vi "Read TDMS.vi"(6 "Append Index":i32, 8 "error in (no error)":errorcluster, 11 "path":path) -> (0 "error out":errorcluster, 1 "Commands":string, 2 "Notes":string, 3 "Data (Dictionary)":T1[](array[typedef]))   [LabVIEW 2016, in "LV-Data.TDMS.lvclass"]
uses:
  LV-Data.TDMS.lvclass
  LV-Data/Typedefs/Dictionary--cluster.ctl
  LV-Data/LV-Data.lvclass
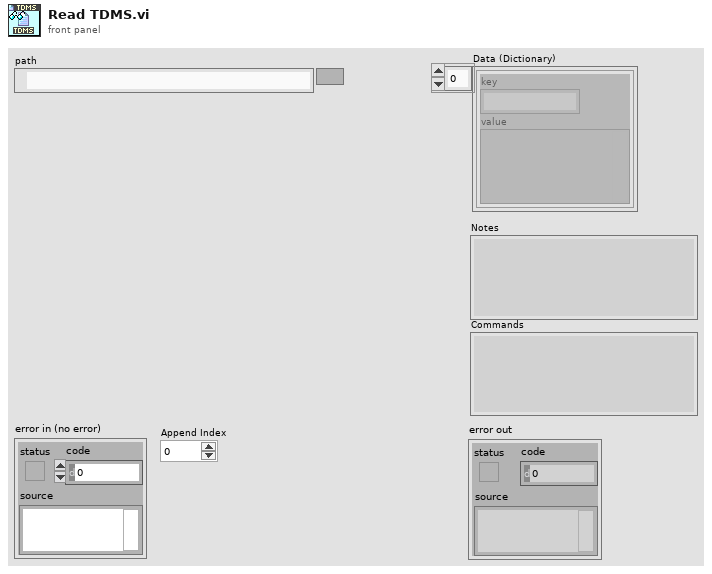
[diagram p1: front panel]
types:
  T1 = typedef "LV-Data.lvclass/Dictionary--cluster.ctl" = cluster{"key":string, "value":variant}
  T2 = enum16{"open", "open or create", "create or replace", "create", "open (read-only)"}
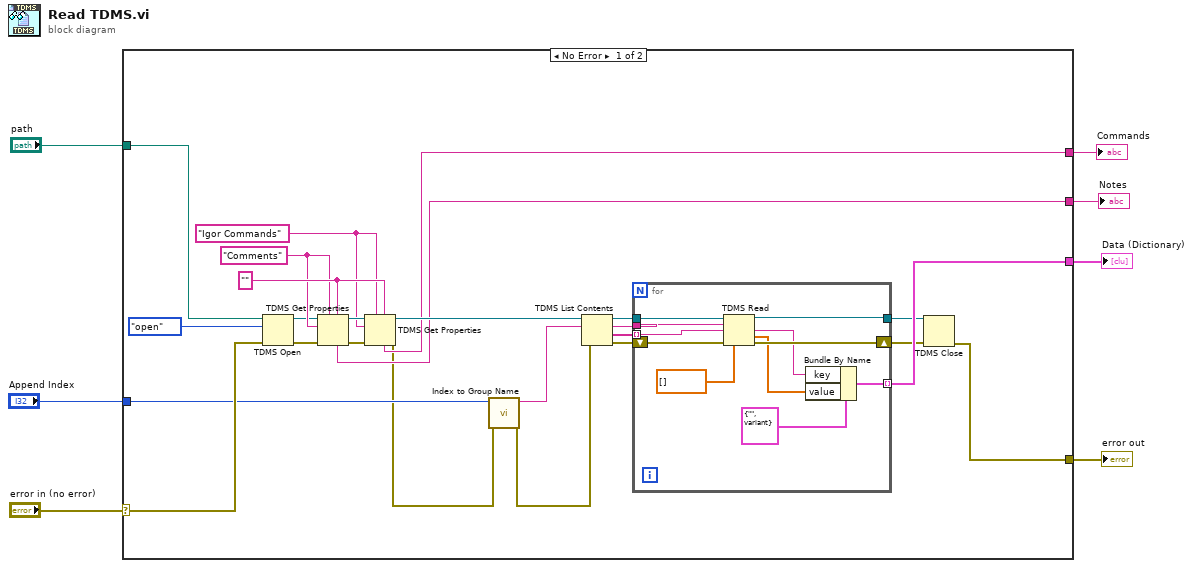
[diagram p0: block diagram]
diagram:
  n1 = case shown="No Error" "error in (no error)" {
    selector: "error in (no error)" -> [w17 w43]
    tunnel: [w12 w43] -> w6
    tunnel: "path" -> [w18 _]
    tunnel: [w22 _] -> w4
    tunnel: [w21 _] -> w3
    tunnel: [w20 _] -> w2
    tunnel: "Append Index" -> [w11 _]
    frame No Error {
      w32 = "" ("attrib name")
      w25 = "Igor Commands" ("attrib name")
      w26 = "Comments" ("attrib name")
      n2 = TDMS Open(8:w17, 10:T2."open" ("operation (0:open)"), 11:w18) -> (0:w15:errorcluster, 3:w16:refnum<k34>)  [unwired: 4 in]
      n3 = TDMS Get Properties(5:w32, 7:w26, 8:w15, 10:w26, 11:w16) -> (0:w29:errorcluster, 3:w30:refnum<k34>, 4:w20:string)  [unwired: 1 in, 3 out]
      n4 = TDMS Get Properties(5:w32, 7:w25, 8:w29, 10:w25, 11:w30) -> (0:w9:errorcluster, 3:w31:refnum<k34>, 4:w21:string)  [unwired: 1 in, 3 out]
      n5 = call "Index to Group Name.vi"("error in (no error)"=w9, "Append Index"=w11) -> ("error out"=w8:errorcluster, "group name in (Untitled)"=w10:string)  [unwired: 8 in]
      n6 = TDMS List Contents(4:w8, 6:w10, 7:w31) -> (0:w27:errorcluster, 1:w23:string[], 2:w24:string, 3:w28:refnum<k34>)
      n7 = for {
        shift-right: [w39] -> w13
        shift-left: w27 -> [w42]
        tunnel: w23 -> [w34] mode=indexing
        tunnel: w24 -> [w38]
        tunnel: [w37] -> w22 mode=indexing
        tunnel: w28 -> [w40]
        tunnel: [w41] -> w14
        n8 = TDMS Read(0:w40, 5:w38, 7:w34, 11:w42, 12:dbl[] [] ("array type (2D Dbl)")) -> (4:w41:refnum<k34>, 10:w33:dbl[], 15:w39:errorcluster)  [unwired: 3 in, 3 out]
        n9 = Bundle By Name(cluster=T1 {"key"="", "value"=variant} ("key-value"), "key"=w34, "value"=w33) -> (w37:T1)
      }
      n10 = TDMS Close(8:w13, 11:w14) -> (0:w12:errorcluster)  [unwired: 1 out]
    }
    frame Error {
    }
  }
  "error out" <- w6
  "Data (Dictionary)" <- w4
  "Commands" <- w3
  "Notes" <- w2
